vi "Swap Array Elements.vi"(9 "y":i32, 10 "x":i32, 11 "unswapped array":string[](array[string])) -> (3 "swapped array":string[](array[string]))   [LabVIEW 2014, in "NIPM_API.lvlib"]
doc: "Swap array elements at indices X and Y.\n\nINPUT(s)\n<B>Unswapped array</B>: 1D string array\n<B>x</B>: index of element to swap with the element at index <B>Y</B> in <B>unswapped array</B>\n<B>y</B>: index of element to swap with the element at index <B>x</B> in <B>unswapped array</B>\n\nOUTPUT(s)\n<B>Swapped array</B>: Returns 1D string array with swapped elements"
uses:
  NIPM_API.lvlib
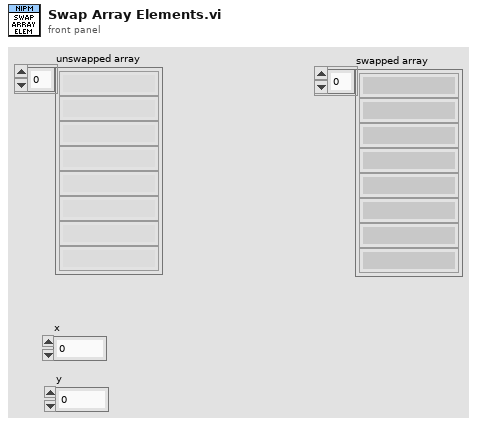
[diagram p1: front panel]
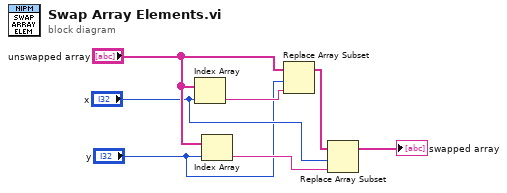
[diagram p0: block diagram]
diagram:
  n1 = Index Array(array="unswapped array", index="x") -> (element=w6:string)
  n2 = Index Array(array="unswapped array", index="y") -> (element=w5:string)
  n3 = Replace Array Subset(array="unswapped array", new element=w6, index="y") -> (w1:string[])
  n4 = Replace Array Subset(array=w1, new element=w5, index="x") -> (→"swapped array":string[])
